vi "omni1.vi"   [LabVIEW 2010, in "Omni2013.lvrbt"]
uses:
  Omni2013.lvrbt
  <vilib>/NXT/NXTIO Xnodes/AddressXNode/NXTIOAddress.xnode
  <vilib>/NXT/Subs/MotorXNode.DC Motor Type.ctl
  <vilib>/NXT/Subs/MotorXNode.2DCMotor.ctl
  <vilib>/NXT/Subs/LVHSConnector.ctl
  <vilib>/NXT/NXTIO Xnodes/NXTIOXNode/NXTIO.xnode
  <vilib>/FTC/FTC Read Controller Packet.vi
  <vilib>/FTC/FTC Read Button States.vi
  <vilib>/NXT/NXTIO Xnodes/NXTIONodeSubVIs/TETRIX IO Move DC Motors.vi
panel:
  # "This VI was generated based on your configuration in the Remote Control Editor. You may modify the code as needed for your robot. To test this program for an FTC match, return to the Remote Control Editor, select the \"Run Program\" tab, and choose \"FTC Game\"."
types:
  T1 = typedef "LVHSConnector.ctl" = cluster{"Hardware":string, "Flattened String":string}
  T2 = typedef "FTC ControllerState.ctl" = cluster{"Left X":i8, "Left Y":i8, "Right X":i8, "Right Y":i8, "Button Encoding 9-12":u8, "Button Encoding 1-8":u8, "POV":T3}
  T3 = typedef "FTC POVState.ctl" = i8
  T4 = typedef "FTC ButtonEventType.ctl" = enum16{"Pressed", "Released"}
  T5 = cluster{"Button ID":enum16{"None", "Button 1", "Button 2", "Button 3", "Button 4", "Button 5", "Button 6", "Button 7", "Button 8", "Button 9", "Button 10", "Button 11", "Button 12", "POV Up", "POV Up Right", "POV Right", "POV Down Right", "POV Down", "POV Down Left", "POV Left", "POV Up Left"}, "Event Type":T4}[]
  T6 = enum16{"None", "Button 1", "Button 2", "Button 3", "Button 4", "Button 5", "Button 6", "Button 7", "Button 8", "Button 9", "Button 10", "Button 11", "Button 12", "POV Up", "POV Up Right", "POV Right", "POV Down Right", "POV Down", "POV Down Left", "POV Left", "POV Up Left"}
  T7 = typedef "MotorXNode.DC Motor Type.ctl" = enum16{"DC Motor"}
  T8 = cluster{"DC Motor":T7, "Address":i16, "Address":i16}
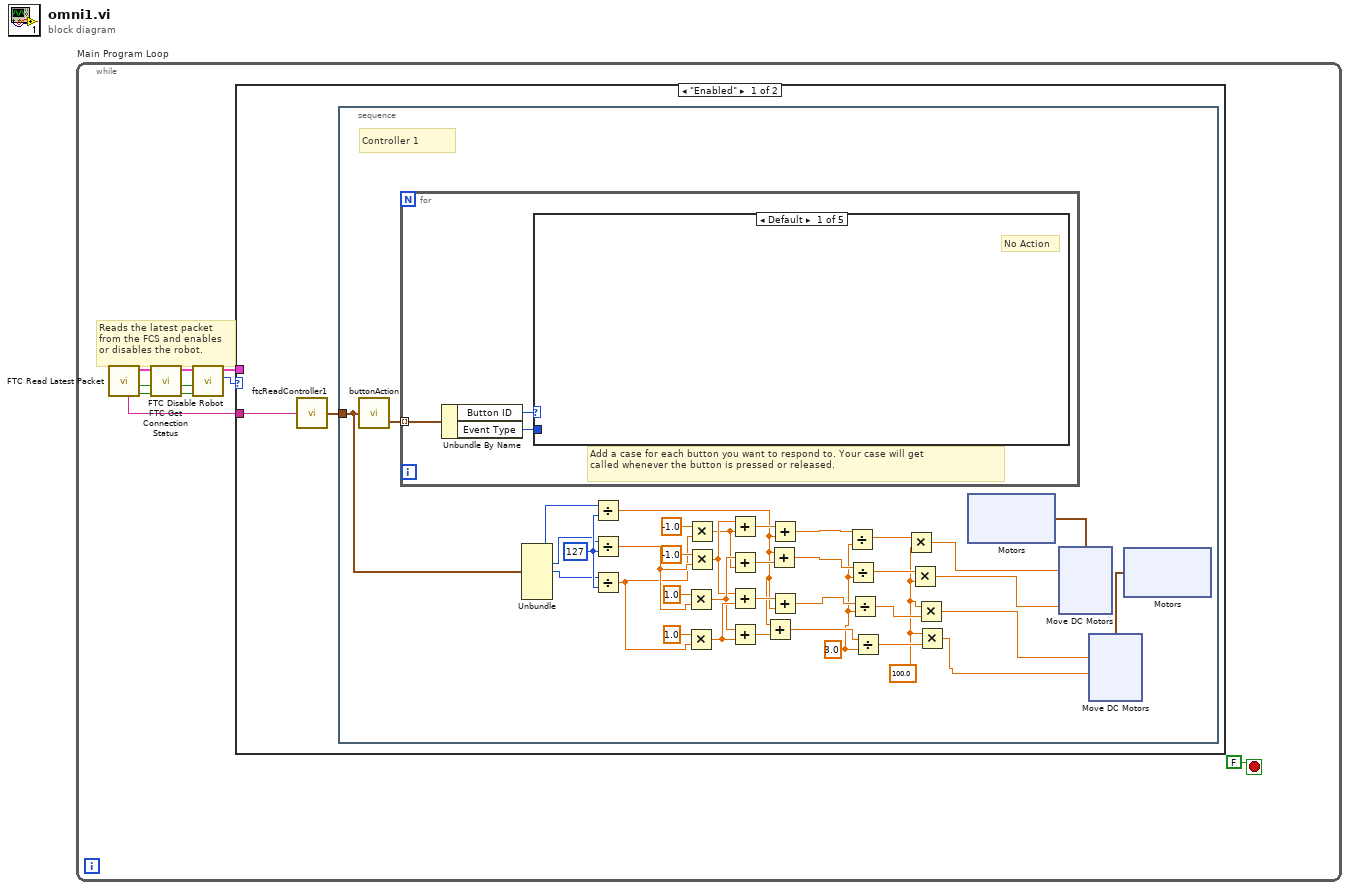
[diagram p0: block diagram]
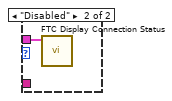
[diagram p6: hidden frame]
diagram:
  n1 = while "Main Program Loop" {
    stop <- FALSE stop-if-true
    # "Reads the latest packet\nfrom the FCS and enables\nor disables the robot."
    n2 = call <vilib>:"FTC Read Latest Packet.vi"() -> ("Packet Received?"=w8:bool, "Stopped?"=w5:bool, "NXT"=w7:T1, "Controller 1"=w9:string)  [unwired: 6 in, 2 out]
    n3 = call <vilib>:"FTC Get Connection Status.vi"("Packet Received?"=w8, "Stopped?"=w5, "NXT"=w7) -> ("Online?"=w2:bool, "Stopped?"=w3:bool, "NXT"=w4:T1)  [unwired: 5 in]
    n4 = call <vilib>:"FTC Disable Robot.vi"("Online?"=w2, "Stopped?"=w3, "NXT"=w4) -> ("Enabled?"=w6:enum16{"Disabled", "Enabled"}, "NXT"=w1:T1)  [unwired: 3 in]
    n5 = case "disableCase" shown="\"Enabled\"" w6 {
      tunnel: w9 -> [w12 _]
      tunnel: w1 -> [_ w75]
      frame "Enabled" {
        n6 = call "ftcReadController1"("Packet"=w12) -> ("Controller State"=w11:T2)  [unwired: 4 in]
        n7 = stacked-sequence "controller1Actions" {
          tunnel: w11 -> [w48]
          frame #0 {
            w19 = 100.0 ("y")
            w24 = 3.0 ("y")
            w46 = i8 127 ("y")
            # "Controller 1"
            n8 = call "buttonAction"("Controller State"=w48) -> ("Button Events"=w49:T5)  [unwired: 2 in, 1 out]
            n9 = for "buttonAction" {
              tunnel: w49 -> [w72] mode=indexing
              # "Add a case for each button you want to respond to. Your case will get \ncalled whenever the button is pressed or released."
              n10 = Unbundle By Name(w72) -> ("Button ID"=w74:T6, "Event Type"=w73:T4)
              n11 = case "EventCase1" shown="Default" w74 {
                tunnel: w73 -> [_ _ _ _ _]
                frame Default {
                  # "No Action"
                }
                frame "Button 5" {
                }
                frame "Button 6" {
                }
                frame "Button 7" {
                }
                frame "Button 8" {
                }
              }
            }
            n12 = Unbundle(w48) -> ("Left X"=w47:i8, "Right X"=w44:i8, "Right Y"=w45:i8)  [unwired: 4 out]
            n13 = Divide(x=w47, y=w46) -> (x/y=w26:dbl)
            n14 = Divide(x=w44, y=w46) -> (x/y=w41:dbl)
            n15 = Divide(x=w45, y=w46) -> (x/y=w38:dbl)
            n16 = Multiply(x=1.0, y=w41) -> (x*y=w36:dbl)
            n17 = Multiply(x=1.0, y=w38) -> (x*y=w37:dbl)
            n18 = Multiply(x=-1.0, y=w38) -> (x*y=w34:dbl)
            n19 = Multiply(x=-1.0, y=w41) -> (x*y=w35:dbl)
            n20 = Add(x=w35, y=w34) -> (x+y=w33:dbl)
            n21 = Add(x=w36, y=w34) -> (x+y=w32:dbl)
            n22 = Add(x=w35, y=w37) -> (x+y=w30:dbl)
            n23 = Add(x=w36, y=w37) -> (x+y=w31:dbl)
            n24 = Add(x=w26, y=w31) -> (x+y=w25:dbl)
            n25 = Add(x=w26, y=w32) -> (x+y=w28:dbl)
            n26 = Add(x=w33, y=w26) -> (x+y=w27:dbl)
            n27 = Add(x=w30, y=w26) -> (x+y=w29:dbl)
            n28 = Divide(x=w27, y=w24) -> (x/y=w23:dbl)
            n29 = Divide(x=w28, y=w24) -> (x/y=w22:dbl)
            n30 = Divide(x=w29, y=w24) -> (x/y=w21:dbl)
            n31 = Divide(x=w25, y=w24) -> (x/y=w20:dbl)
            n32 = Multiply(x=w23, y=w19) -> (x*y=w18:dbl)
            n33 = Multiply(x=w22, y=w19) -> (x*y=w16:dbl)
            n34 = Multiply(x=w19, y=w21) -> (x*y=w14:dbl)
            n35 = Multiply(x=w19, y=w20) -> (x*y=w13:dbl)
            n36 = xnode "Motors"() -> ("DC Motor"=w17:T8)
            n37 = xnode "Move DC Motors"("Power/Speed 2"=w16, "Power/Speed 1"=w18, "Motors"=w17) -> ()  [unwired: 1 in, 1 out]
            n38 = xnode "Motors"() -> ("DC Motor"=w15:T8)
            n39 = xnode "Move DC Motors"("Power/Speed 2"=w13, "Power/Speed 1"=w14, "Motors"=w15) -> ()  [unwired: 1 in, 1 out]
          }
        }
      }
      frame "Disabled" {
        n40 = call <vilib>:"FTC Display Connection Status.vi"("NXT"=w75) -> ()  [unwired: 10 in, 1 out]
      }
    }
  }
